vi "PAN_ParseCmd.vi"(10 "cmd in":string) -> (2 "cmd ref out":string)   [LabVIEW 2016]
uses:
  Modules/DBSHAND/private/vis/DatabaseHand_Element_Get(string).vi
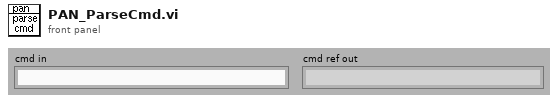
[diagram p1: front panel]
types:
  T1 = typedef "DatabaseHand_RefNum.ctl" = refnum<vi>
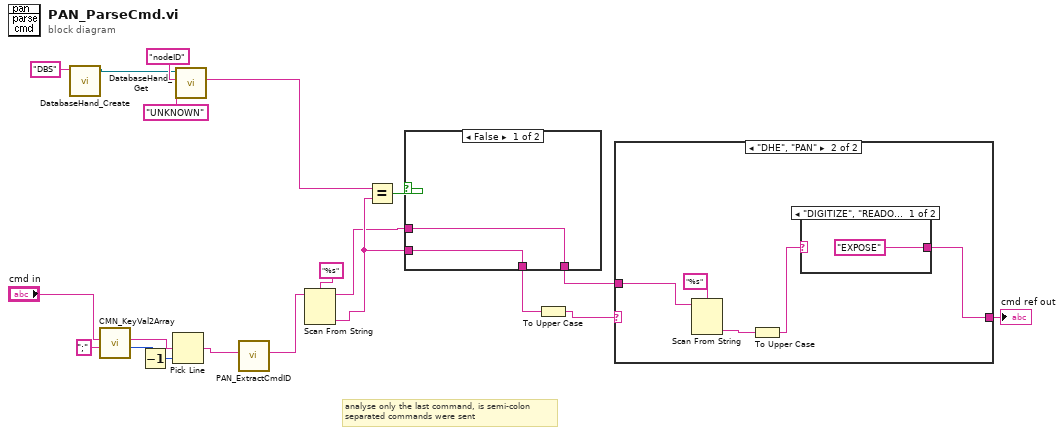
[diagram p0: block diagram]
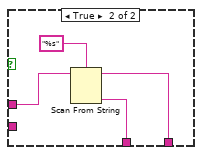
[diagram p2: hidden frame]
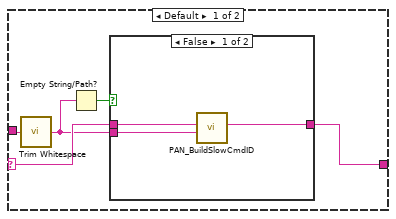
[diagram p3: hidden frame]
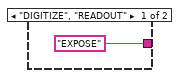
[diagram p5: hidden frame]
diagram:
  # "analyse only the last command, is semi-colon\nseparated commands were sent"
  n1 = call "DatabaseHand_Create.vi"("Name"="DBS") -> ("Database RefNum out"=w10:T1)  [unwired: 1 in, 9 out]
  n2 = call "CMN_KeyVal2Array.vi"("separator"=";", "command in"="cmd in") -> ("number of commands"=w15:i32, "commands out"=w16:string)  [unwired: 1 in, 6 out]
  n3 = Decrement(x=w15) -> (x-1=w14:i32)
  n4 = Pick Line(multi-line string=w16, line index=w14) -> (output string=w2:string)  [unwired: 1 out]
  n5 = call-poly "DatabaseHand_Get.vi"("default value"="UNKNOWN", "name"="nodeID", "Database RefNum in"=w10) -> ("value"=w8:string)  [unwired: 2 in, 6 out]
  n6 = call "PAN_ExtractCmdID.vi"("command in"=w2) -> ("cmd out"=w1:string)  [unwired: 10 out]
  n7 = Scan From String(format string="%s", input string=w1) -> (remaining string=w4:string, output 1=w6:string)  [unwired: 2 in, 3 out]
  n8 = Equal?(x=w8, y=w6) -> (x = y?=w7:bool)
  n9 = case shown="False" w7 {
    tunnel: w6 -> [w22 _]
    tunnel: w4 -> [w21 w26]
    tunnel: [w22 w24] -> w5
    tunnel: [w21 w23] -> w3
    frame False {
    }
    frame True {
      n10 = Scan From String(format string="%s", input string=w26) -> (remaining string=w23:string, output 1=w24:string)  [unwired: 2 in, 3 out]
    }
  }
  n11 = To Upper Case(1:w5) -> (0:w19:string)
  n12 = case shown="\"DHE\", \"PAN\"" w19 {
    selector: w19 -> [w30 _]
    tunnel: [w29 w39] -> w18
    tunnel: w3 -> [w31 w41]
    frame Default {
      n13 = call <vilib>:"Trim Whitespace.vi"("string"=w31) -> ("trimmed string"=w28:string)  [unwired: 1 in]
      n14 = Empty String/Path?(string/path=w28) -> (empty?=w27:bool)
      n15 = case shown="False" w27 {
        tunnel: w28 -> [w34 _]
        tunnel: w30 -> [w33 w36]
        tunnel: [w32 w35] -> w29
        frame False {
          n16 = call "PAN_BuildSlowCmdID.vi"("Command"=w34, "caller"=w33) -> ("cmdID"=w32:string)  [unwired: 1 in, 8 out]
        }
        frame True {
          n17 = case shown="Default" w36 {
            selector: w36 -> [_ w38]
            tunnel: ["EXPOSE" w38] -> w35
            frame "DIGITIZE", "READOUT" {
            }
            frame Default {
            }
          }
        }
      }
    }
    frame "DHE", "PAN" {
      n18 = Scan From String(format string="%s", input string=w41) -> (output 1=w42:string)  [unwired: 2 in, 4 out]
      n19 = To Upper Case(1:w42) -> (0:w40:string)
      n20 = case shown="\"DIGITIZE\", \"READOUT\"" w40 {
        selector: w40 -> [_ w45]
        tunnel: ["EXPOSE" w45] -> w39
        frame "DIGITIZE", "READOUT" {
        }
        frame Default {
        }
      }
    }
  }
  "cmd ref out" <- w18
